vi "State_Machine.vi"(0 "Process_REF":string, 1 "Emergency":bool, 2 "Start Process":bool, 3 "Initialized":bool, 4 "Input Validated":bool, 5 "error in (no error)":errorcluster, 6 "Action":enum16{""}(ring), 7 "Running Done":bool, 9 "Process Complete":bool, 11 "Progressing":bool, 12 "Reset":bool, 13 "Powering Down":bool) -> (14 "Path Out":path, 15 "State":dbl, 16 "State String":string, 19 "error out":errorcluster)   [LabVIEW 2018]
panel:
  in  "Empty 2":bool
  in  "Empty1":bool
  out "_C_Powering_Down":bool
  out "_C_Empty_2":bool
  out "_C_Start_Process":bool
  out "_C_Empty_1":bool
  out "_C_Progressing":bool
  out "_C_Process Complete":bool
  out "_C_Running_Done":bool
  out "_C_Input_Validated":bool
  out "_C_Initialized":bool
  out "_C_emergency":bool
  out "_Powering Down":bool
  out "_Progressing Stage":bool
  out "_Completing Stage":bool
  out "_Running Stage":bool
  out "_Validating Input":bool
  out "_Initializing":bool
  out "_Idle":bool
  out "_Emergency":bool
  out "_Current_State":dbl
  # "~~~STATE MACHINE OUTPUT KEY~~~\n~~~ 1x Numeric & 1x Boolean ~~~\n(neg) - Emergency\n   All negative values\n(max) - Powering Down\n   All values above max\n0 -Idle\n1 - Initializing\n2 - Validating Input\n3 - Running Stage\n4 - Completing Stage\n5 - Progressing Stage\nBoolean - (T/F) Emergency Status"
  # "~~~INPUT CONDITIONS KEY~~~\n~~~ x10 Boolean Values~~~\n1 - Emergency\n2 - Start Process\n3 - Initialized\n4 - Input Validated\n5 - Running Done\n6 - Process Complete\n7 - Progressing (To next stage)\n8 - (Empty 1)\n9 - (Empty 2)\n10 - Powering Down"
  # "Local Variables (Used For Debugging)"
  # "State Lights"
  # "Condition Lights"
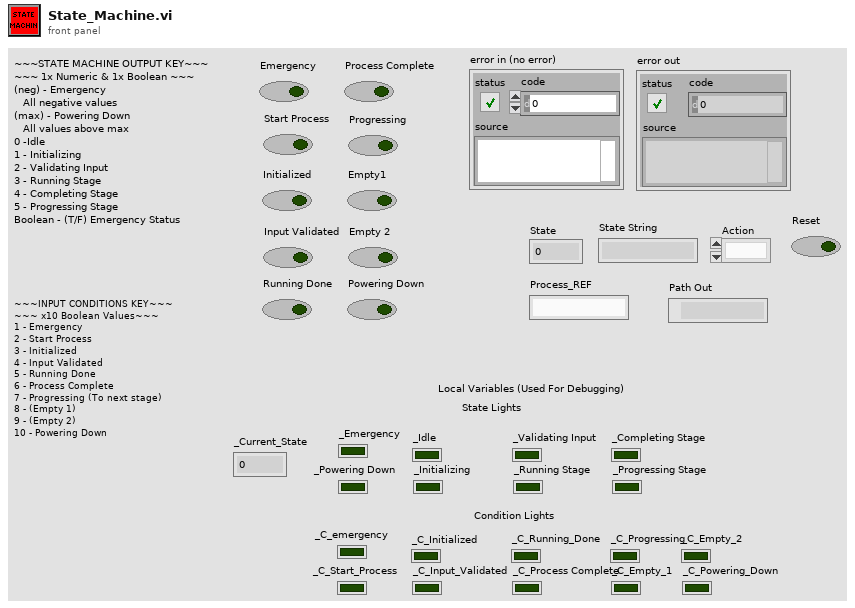
[diagram p1: front panel]
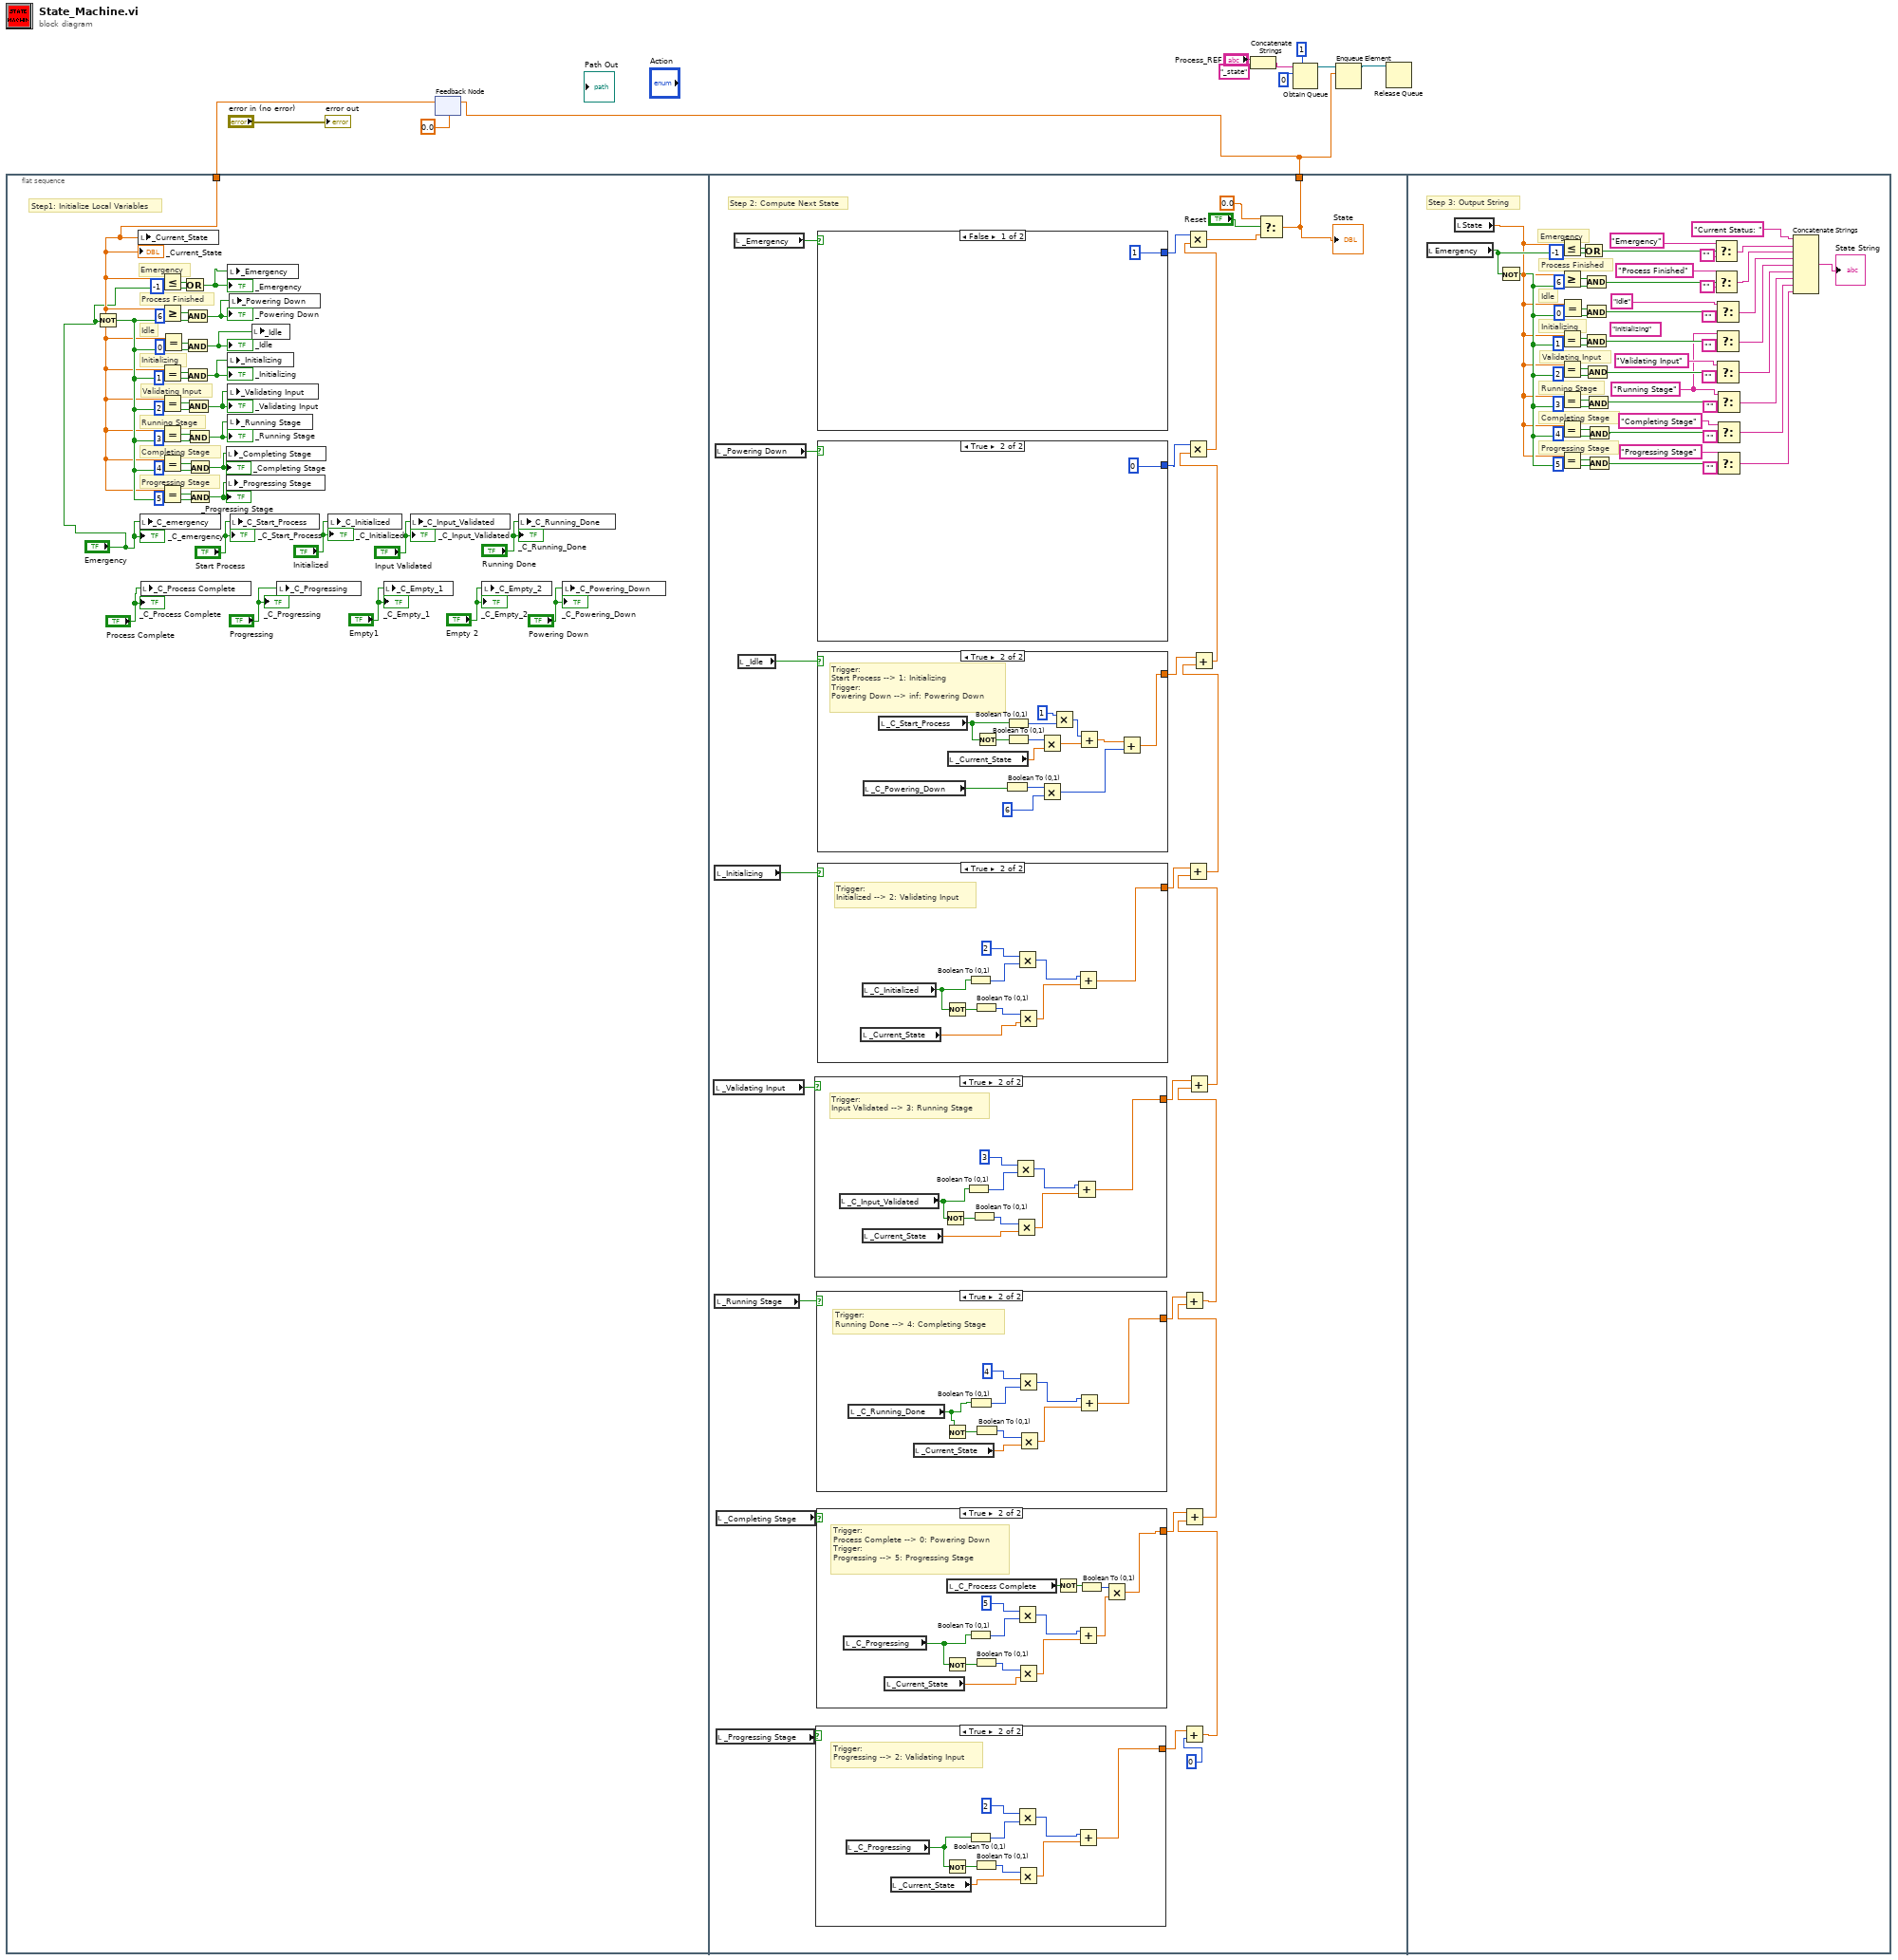
[diagram p0: block diagram]
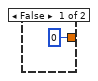
[diagram p2: hidden frame]
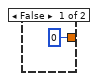
[diagram p3: hidden frame]
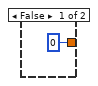
[diagram p4: hidden frame]
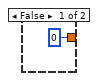
[diagram p5: hidden frame]
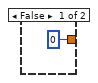
[diagram p6: hidden frame]
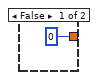
[diagram p7: hidden frame]
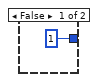
[diagram p8: hidden frame]
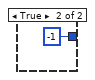
[diagram p9: hidden frame]
diagram:
  n1 = flat-sequence {
    tunnel: w10 -> [w22]
    tunnel: [w48] -> w3
    frame #0 {
      # "Step1: Initialize Local Variables"
      # "Emergency"
      # "Process Finished"
      # "Progressing Stage"
      # "Completing Stage"
      # "Running Stage"
      # "Validating Input"
      # "Initializing"
      # "Idle"
      n2 = Not(x="Emergency") -> (.not. x?=w36:bool)
      n3 = local write "_Current_State"(w22) -> ()
      n4 = local write "_C_emergency"("Emergency") -> ()
      n5 = local write "_C_Process Complete"("Process Complete") -> ()
      n6 = Less Or Equal?(x=w22, y=-1) -> (x <= y?=w25:bool)
      n7 = Greater Or Equal?(x=w22, y=6) -> (x >= y?=w23:bool)
      n8 = Equal?(x=w22, y=1) -> (x = y?=w38:bool)
      n9 = Equal?(x=w22, y=2) -> (x = y?=w39:bool)
      n10 = Equal?(x=w22, y=3) -> (x = y?=w40:bool)
      n11 = Equal?(x=w22, y=4) -> (x = y?=w41:bool)
      n12 = Equal?(x=w22, y=5) -> (x = y?=w27:bool)
      n13 = Equal?(x=w22, y=0) -> (x = y?=w37:bool)
      n14 = Or(x=w25, y="Emergency") -> (x .or. y?=w35:bool)
      "_Emergency" <- w35
      n15 = And(x=w23, y=w36) -> (x .and. y?=w34:bool)
      "_Powering Down" <- w34
      n16 = And(x=w37, y=w36) -> (x .and. y?=w33:bool)
      "_Idle" <- w33
      n17 = And(x=w38, y=w36) -> (x .and. y?=w32:bool)
      "_Initializing" <- w32
      n18 = And(x=w39, y=w36) -> (x .and. y?=w31:bool)
      "_Validating Input" <- w31
      n19 = And(x=w40, y=w36) -> (x .and. y?=w30:bool)
      "_Running Stage" <- w30
      n20 = And(x=w41, y=w36) -> (x .and. y?=w29:bool)
      "_Completing Stage" <- w29
      n21 = And(x=w27, y=w36) -> (x .and. y?=w28:bool)
      "_Progressing Stage" <- w28
      n22 = local write "_Completing Stage"(w29) -> ()
      n23 = local write "_Progressing Stage"(w28) -> ()
      n24 = local write "_Emergency"(w35) -> ()
      n25 = local write "_Initializing"(w32) -> ()
      n26 = local write "_Validating Input"(w31) -> ()
      n27 = local write "_Running Stage"(w30) -> ()
      n28 = local write "_Powering Down"(w34) -> ()
      n29 = local write "_C_Start_Process"("Start Process") -> ()
      n30 = local write "_Idle"(w33) -> ()
      n31 = local write "_C_Progressing"("Progressing") -> ()
      n32 = local write "_C_Initialized"("Initialized") -> ()
      n33 = local write "_C_Empty_1"("Empty1") -> ()
      n34 = local write "_C_Input_Validated"("Input Validated") -> ()
      n35 = local write "_C_Empty_2"("Empty 2") -> ()
      n36 = local write "_C_Running_Done"("Running Done") -> ()
      n37 = local write "_C_Powering_Down"("Powering Down") -> ()
      "_Current_State" <- w22
      "_C_emergency" <- "Emergency"
      "_C_Initialized" <- "Initialized"
      "_C_Input_Validated" <- "Input Validated"
      "_C_Running_Done" <- "Running Done"
      "_C_Process Complete" <- "Process Complete"
      "_C_Progressing" <- "Progressing"
      "_C_Empty_1" <- "Empty1"
      "_C_Start_Process" <- "Start Process"
      "_C_Empty_2" <- "Empty 2"
      "_C_Powering_Down" <- "Powering Down"
    }
    frame #1 {
      # "Step 2: Compute Next State"
      n38 = local read "_Validating Input"() -> (w71:bool)
      n39 = local read "_Initializing"() -> (w72:bool)
      n40 = local read "_Running Stage"() -> (w70:bool)
      n41 = local read "_Powering Down"() -> (w74:bool)
      n42 = local read "_Completing Stage"() -> (w69:bool)
      n43 = local read "_Progressing Stage"() -> (w68:bool)
      n44 = local read "_Emergency"() -> (w75:bool)
      n45 = local read "_Idle"() -> (w73:bool)
      n46 = case shown="True" w71 {
        tunnel: [0 w111] -> w58
        frame False {
        }
        frame True {
          # "Trigger:\nInput Validated --> 3: Running Stage"
          n47 = local read "_C_Input_Validated"() -> (w113:bool)
          n48 = local read "_Current_State"() -> (w112:dbl)
          n49 = Not(x=w113) -> (.not. x?=w119:bool)
          n50 = Boolean To (0,1)(Boolean=w113) -> (0, 1=w117:i16)
          n51 = Boolean To (0,1)(Boolean=w119) -> (0, 1=w116:i16)
          n52 = Multiply(x=3, y=w117) -> (x*y=w114:i32)
          n53 = Multiply(x=w116, y=w112) -> (x*y=w115:dbl)
          n54 = Add(x=w114, y=w115) -> (x+y=w111:dbl)
        }
      }
      n55 = case shown="True" w68 {
        tunnel: [0 w77] -> w55
        frame False {
        }
        frame True {
          # "Trigger:\nProgressing --> 2: Validating Input"
          n56 = local read "_C_Progressing"() -> (w79:bool)
          n57 = local read "_Current_State"() -> (w78:dbl)
          n58 = Not(x=w79) -> (.not. x?=w85:bool)
          n59 = Boolean To (0,1)(Boolean=w79) -> (0, 1=w83:i16)
          n60 = Boolean To (0,1)(Boolean=w85) -> (0, 1=w82:i16)
          n61 = Multiply(x=2, y=w83) -> (x*y=w80:i32)
          n62 = Multiply(x=w82, y=w78) -> (x*y=w81:dbl)
          n63 = Add(x=w80, y=w81) -> (x+y=w77:dbl)
        }
      }
      n64 = case shown="True" w70 {
        tunnel: [0 w101] -> w57
        frame False {
        }
        frame True {
          # "Trigger:\nRunning Done --> 4: Completing Stage"
          n65 = local read "_C_Running_Done"() -> (w103:bool)
          n66 = local read "_Current_State"() -> (w102:dbl)
          n67 = Not(x=w103) -> (.not. x?=w109:bool)
          n68 = Boolean To (0,1)(Boolean=w103) -> (0, 1=w107:i16)
          n69 = Boolean To (0,1)(Boolean=w109) -> (0, 1=w106:i16)
          n70 = Multiply(x=4, y=w107) -> (x*y=w104:i32)
          n71 = Multiply(x=w106, y=w102) -> (x*y=w105:dbl)
          n72 = Add(x=w104, y=w105) -> (x+y=w101:dbl)
        }
      }
      n73 = case shown="True" w69 {
        tunnel: [0 w92] -> w56
        frame False {
        }
        frame True {
          # "Trigger:\nProcess Complete --> 0: Powering Down\nTrigger:\nProgressing --> 5: Progressing Stage"
          n74 = local read "_C_Progressing"() -> (w91:bool)
          n75 = local read "_Current_State"() -> (w90:dbl)
          n76 = Not(x=w91) -> (.not. x?=w99:bool)
          n77 = local read "_C_Process Complete"() -> (w89:bool)
          n78 = Boolean To (0,1)(Boolean=w91) -> (0, 1=w97:i16)
          n79 = Boolean To (0,1)(Boolean=w99) -> (0, 1=w96:i16)
          n80 = Multiply(x=5, y=w97) -> (x*y=w94:i32)
          n81 = Multiply(x=w96, y=w90) -> (x*y=w95:dbl)
          n82 = Not(x=w89) -> (.not. x?=w88:bool)
          n83 = Add(x=w94, y=w95) -> (x+y=w93:dbl)
          n84 = Boolean To (0,1)(Boolean=w88) -> (0, 1=w87:i16)
          n85 = Multiply(x=w87, y=w93) -> (x*y=w92:dbl)
        }
      }
      n86 = case shown="False" w75 {
        tunnel: [1 -1] -> w67
        frame False {
        }
        frame True {
        }
      }
      n87 = case shown="True" w74 {
        tunnel: [1 0] -> w52
        frame False {
        }
        frame True {
        }
      }
      n88 = case shown="True" w73 {
        tunnel: [0 w136] -> w60
        frame False {
        }
        frame True {
          # "Trigger:\nStart Process --> 1: Initializing\nTrigger:\nPowering Down --> inf: Powering Down"
          n89 = local read "_C_Powering_Down"() -> (w134:bool)
          n90 = local read "_C_Start_Process"() -> (w143:bool)
          n91 = local read "_Current_State"() -> (w140:dbl)
          n92 = Not(x=w143) -> (.not. x?=w144:bool)
          n93 = Boolean To (0,1)(Boolean=w134) -> (0, 1=w133:i16)
          n94 = Boolean To (0,1)(Boolean=w143) -> (0, 1=w141:i16)
          n95 = Boolean To (0,1)(Boolean=w144) -> (0, 1=w139:i16)
          n96 = Multiply(x=w139, y=w140) -> (x*y=w138:dbl)
          n97 = Multiply(x=w133, y=6) -> (x*y=w131:i32)
          n98 = Multiply(x=1, y=w141) -> (x*y=w137:i32)
          n99 = Add(x=w137, y=w138) -> (x+y=w135:dbl)
          n100 = Add(x=w135, y=w131) -> (x+y=w136:dbl)
        }
      }
      n101 = case shown="True" w72 {
        tunnel: [0 w121] -> w59
        frame False {
        }
        frame True {
          # "Trigger:\nInitialized --> 2: Validating Input"
          n102 = local read "_Current_State"() -> (w123:dbl)
          n103 = local read "_C_Initialized"() -> (w122:bool)
          n104 = Not(x=w122) -> (.not. x?=w129:bool)
          n105 = Boolean To (0,1)(Boolean=w122) -> (0, 1=w127:i16)
          n106 = Boolean To (0,1)(Boolean=w129) -> (0, 1=w126:i16)
          n107 = Multiply(x=2, y=w127) -> (x*y=w124:i32)
          n108 = Multiply(x=w126, y=w123) -> (x*y=w125:dbl)
          n109 = Add(x=w124, y=w125) -> (x+y=w121:dbl)
        }
      }
      n110 = Add(x=w55, y=0) -> (x+y=w62:dbl)
      n111 = Add(x=w56, y=w62) -> (x+y=w63:dbl)
      n112 = Add(x=w57, y=w63) -> (x+y=w64:dbl)
      n113 = Add(x=w58, y=w64) -> (x+y=w65:dbl)
      n114 = Add(x=w59, y=w65) -> (x+y=w66:dbl)
      n115 = Add(x=w60, y=w66) -> (x+y=w53:dbl)
      n116 = Multiply(x=w52, y=w53) -> (x*y=w54:dbl)
      n117 = Multiply(x=w67, y=w54) -> (x*y=w51:dbl)
      n118 = Select(t=0.0, s="Reset", f=w51) -> (s? t:f=w48:dbl)
      "State" <- w48
    }
    frame #2 {
      w149 = "Running Stage"
      (unwired) "Initializing"
      # "Emergency"
      # "Process Finished"
      # "Progressing Stage"
      # "Completing Stage"
      # "Running Stage"
      # "Validating Input"
      # "Initializing"
      # "Idle"
      # "Step 3: Output String"
      n119 = local read "Emergency"() -> (w183:bool)
      n120 = local read "State"() -> (w155:dbl)
      n121 = Not(x=w183) -> (.not. x?=w184:bool)
      n122 = Less Or Equal?(x=w155, y=-1) -> (x <= y?=w187:bool)
      n123 = Greater Or Equal?(x=w155, y=6) -> (x >= y?=w185:bool)
      n124 = Equal?(x=w155, y=1) -> (x = y?=w191:bool)
      n125 = Equal?(x=w155, y=2) -> (x = y?=w192:bool)
      n126 = Equal?(x=w155, y=3) -> (x = y?=w193:bool)
      n127 = Equal?(x=w155, y=4) -> (x = y?=w194:bool)
      n128 = Equal?(x=w155, y=5) -> (x = y?=w189:bool)
      n129 = Equal?(x=w155, y=0) -> (x = y?=w190:bool)
      n130 = Or(x=w187, y=w183) -> (x .or. y?=w182:bool)
      n131 = And(x=w185, y=w184) -> (x .and. y?=w179:bool)
      n132 = And(x=w190, y=w184) -> (x .and. y?=w178:bool)
      n133 = And(x=w191, y=w184) -> (x .and. y?=w177:bool)
      n134 = And(x=w192, y=w184) -> (x .and. y?=w176:bool)
      n135 = And(x=w193, y=w184) -> (x .and. y?=w175:bool)
      n136 = And(x=w194, y=w184) -> (x .and. y?=w174:bool)
      n137 = And(x=w189, y=w184) -> (x .and. y?=w173:bool)
      n138 = Select(t="Emergency", s=w182, f="") -> (s? t:f=w151:string)
      n139 = Select(t="Process Finished", s=w179, f="") -> (s? t:f=w152:string)
      n140 = Select(t="Idle", s=w178, f="") -> (s? t:f=w153:string)
      n141 = Select(t=w149, s=w177, f="") -> (s? t:f=w156:string)
      n142 = Select(t="Validating Input", s=w176, f="") -> (s? t:f=w157:string)
      n143 = Select(t=w149, s=w175, f="") -> (s? t:f=w158:string)
      n144 = Select(t="Completing Stage", s=w174, f="") -> (s? t:f=w159:string)
      n145 = Select(t="Progressing Stage", s=w173, f="") -> (s? t:f=w160:string)
      n146 = Concatenate Strings("Current Status: ", w151, w152, w153, w156, w157, w158, w159, w160) -> (→"State String":string)
    }
  }
  n147 = feedback #1(0.0) -> (w10:dbl)
  n148 = feedback-in #1(w3) -> ()
  n149 = Concatenate Strings("Process_REF", "_state") -> (w6:string)
  n150 = Obtain Queue(max queue size (-1, unlimited)=1, name (unnamed)=w6, element data type=0) -> (queue out=w4:refnum<queue>)  [unwired: 2 in, 2 out]
  n151 = Enqueue Element(queue=w4, element=w3) -> (queue out=w1:refnum<queue>)  [unwired: 2 in, 2 out]
  n152 = Release Queue(queue=w1) -> ()  [unwired: 2 in, 3 out]
  "error out" <- "error in (no error)"
